vi "Rysowanie prostej.vi"(1 "Środek":u16[](array[numeric]), 2 "Skalowanie":u32=1 min=1, 3 "Równanie prostej":dbl[](array[numeric]), 4 "picture":picture) -> (0 "new picture":picture)   [LabVIEW 2016]
doc: "To Vi rysuje prostą zadaną równaniem względem zadanego środka i z podanym przeskalowaniem"
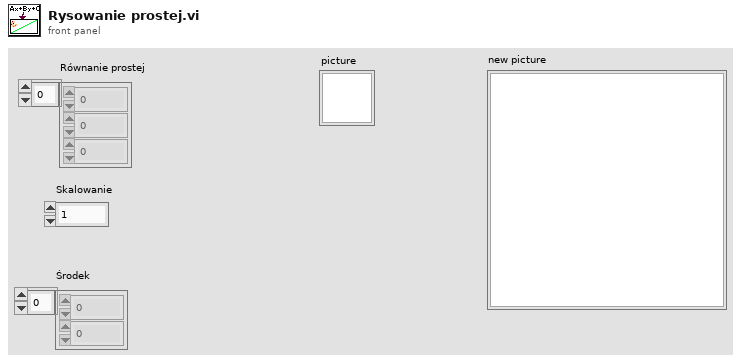
[diagram p1: front panel]
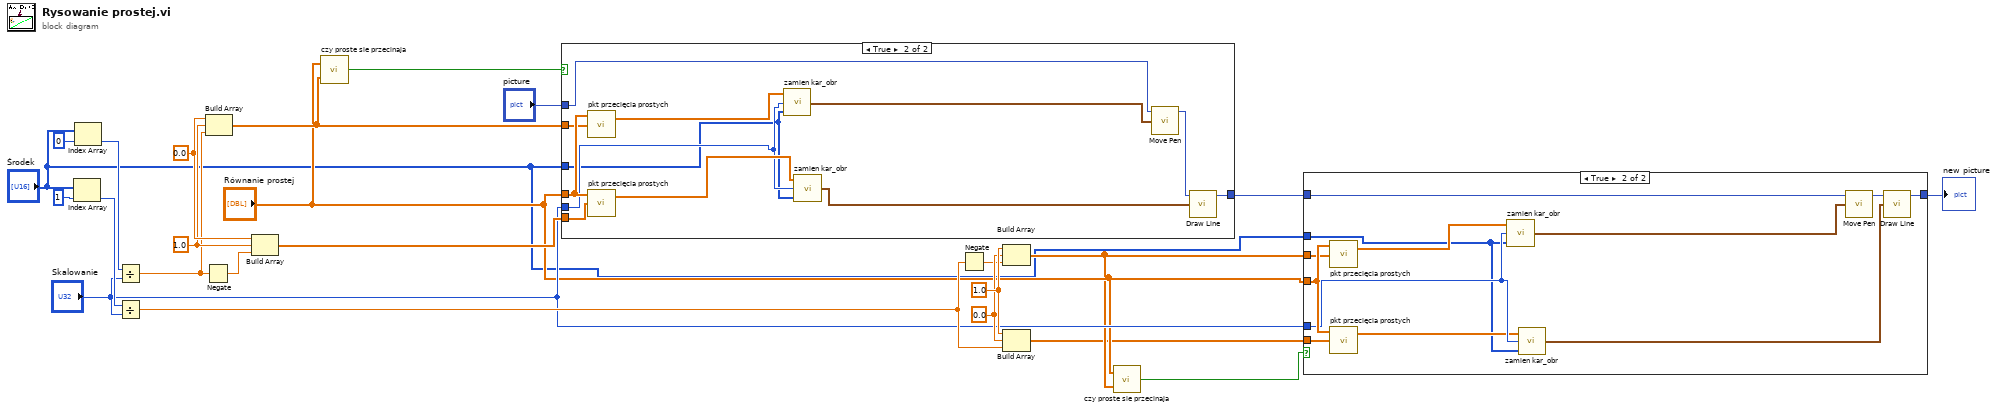
[diagram p0: block diagram]
diagram:
  w18 = 0.0 ("element")
  w19 = 1.0 ("element")
  w20 = 1.0 ("element")
  w21 = 0.0 ("element")
  n1 = Index Array(array="Środek", index=1) -> (element=w22:u16)
  n2 = Index Array(array="Środek", index=0) -> (element=w6:u16)
  n3 = Divide(x=w6, y="Skalowanie") -> (x/y=w17:dbl)
  n4 = Divide(x=w22, y="Skalowanie") -> (x/y=w14:dbl)
  n5 = Negate(x=w17) -> (-x=w16:dbl)
  n6 = Build Array(w21, w20, w17) -> (w12:dbl[])
  n7 = Build Array(w21, w20, w16) -> (w11:dbl[])
  n8 = call "czy proste sie przecinaja.vi"("Równanie Prostej 2"=w12, "Równanie Prostej 1"="Równanie prostej") -> ("x != 0?"=w13:bool)
  n9 = case shown="True" w13 {
    tunnel: "Równanie prostej" -> [_ w37]
    tunnel: w12 -> [_ w36]
    tunnel: w11 -> [_ w35]
    tunnel: "Skalowanie" -> [_ w28]
    tunnel: "picture" -> [w25 w34]
    tunnel: [w25 w32] -> w9
    tunnel: "Środek" -> [_ w27]
    frame False {
    }
    frame True {
      n10 = call "pkt przecięcia prostych.vi"("Równanie Prostej 2"=w36, "Równanie Prostej 1"=w37) -> ("subarray"=w31:dbl[])  [unwired: 1 in, 1 out]
      n11 = call "pkt przecięcia prostych.vi"("Równanie Prostej 2"=w35, "Równanie Prostej 1"=w37) -> ("subarray"=w29:dbl[])  [unwired: 1 in, 1 out]
      n12 = call "zamien kar_obr.vi"("Środek"=w27, "Skalowanie"=w28, "Pkt"=w31) -> ("pkt we wsp obrazu"=w30:cluster{i16, i16})
      n13 = call "zamien kar_obr.vi"("Środek"=w27, "Skalowanie"=w28, "Pkt"=w29) -> ("pkt we wsp obrazu"=w26:cluster{i16, i16})
      n14 = call <vilib>:"Move Pen.vi"("new position"=w30, "picture"=w34) -> ("new picture"=w33:picture)  [unwired: 3 in]
      n15 = call <vilib>:"Draw Line.vi"("picture"=w33, "end point"=w26) -> ("new picture"=w32:picture)  [unwired: 7 in]
    }
  }
  n16 = Negate(x=w14) -> (-x=w15:dbl)
  n17 = Build Array(w19, w18, w15) -> (w3:dbl[])
  n18 = Build Array(w19, w18, w14) -> (w2:dbl[])
  n19 = call "czy proste sie przecinaja.vi"("Równanie Prostej 2"=w3, "Równanie Prostej 1"="Równanie prostej") -> ("x != 0?"=w4:bool)
  n20 = case shown="True" w4 {
    tunnel: "Równanie prostej" -> [_ w50]
    tunnel: w3 -> [_ w49]
    tunnel: w2 -> [_ w48]
    tunnel: "Skalowanie" -> [_ w42]
    tunnel: w9 -> [w38 w47]
    tunnel: [w38 w45] -> w8
    tunnel: "Środek" -> [_ w40]
    frame False {
    }
    frame True {
      n21 = call "pkt przecięcia prostych.vi"("Równanie Prostej 2"=w49, "Równanie Prostej 1"=w50) -> ("subarray"=w44:dbl[])  [unwired: 1 in, 1 out]
      n22 = call "pkt przecięcia prostych.vi"("Równanie Prostej 2"=w48, "Równanie Prostej 1"=w50) -> ("subarray"=w41:dbl[])  [unwired: 1 in, 1 out]
      n23 = call "zamien kar_obr.vi"("Środek"=w40, "Skalowanie"=w42, "Pkt"=w44) -> ("pkt we wsp obrazu"=w43:cluster{i16, i16})
      n24 = call "zamien kar_obr.vi"("Środek"=w40, "Skalowanie"=w42, "Pkt"=w41) -> ("pkt we wsp obrazu"=w39:cluster{i16, i16})
      n25 = call <vilib>:"Move Pen.vi"("new position"=w43, "picture"=w47) -> ("new picture"=w46:picture)  [unwired: 3 in]
      n26 = call <vilib>:"Draw Line.vi"("picture"=w46, "end point"=w39) -> ("new picture"=w45:picture)  [unwired: 7 in]
    }
  }
  "new picture" <- w8
